vi "Commands to ITX.vi"(1 "Commands":string) -> (0 "ITX Commands":string)   [LabVIEW 2019, in "ITX Commands.lvclass"]
uses:
  ITX Commands.lvclass
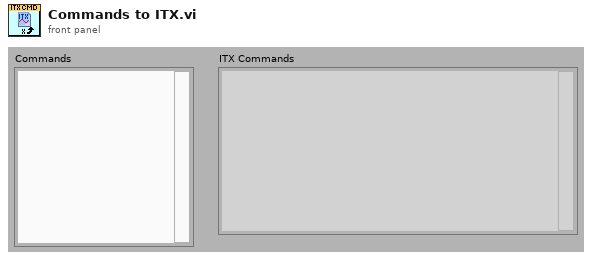
[diagram p1: front panel]
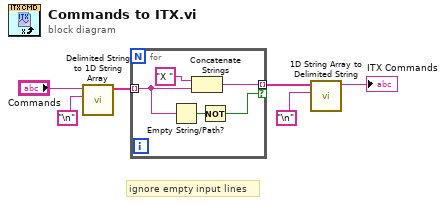
[diagram p0: block diagram]
diagram:
  # "ignore empty input lines"
  n1 = call <vilib>:"Delimited String to 1D String Array.vi"("delimiter"="\n", "delimited string"="Commands") -> ("string array"=w5:string[])  [unwired: 9 in]
  n2 = for {
    tunnel: w5 -> [w9] mode=indexing
    tunnel: [w10] -> w4 mode=indexing if=w7
    n3 = Empty String/Path?(string/path=w9) -> (empty?=w8:bool)
    n4 = Concatenate Strings("X " ("string"), w9) -> (w10:string)
    n5 = Not(x=w8) -> (.not. x?=w7:bool)
  }
  n6 = call <vilib>:"1D String Array to Delimited String.vi"("delimiter"="\n", "string array"=w4) -> ("delimited string"=→"ITX Commands":string)  [unwired: 9 in]
